vi "oa_TV Time Index Angle (1Chan).vi"(0 "pulse positions":dbl[](array[numeric]), 5 "angle intervals":dbl[](array[numeric]), 7 "revolution":i32, 9 "revolution index":i32, 11 "error in (no error)":errorcluster) -> (4 "pulse positions":dbl[](array[numeric]), 6 "angle":dbl[](array[numeric]), 15 "error out":errorcluster)   [LabVIEW 2017, in "SoundVib_Torsional.lvlib"]
uses:
  <vilib>/addons/Sound and Vibration/Order Analysis/Torsional Vibration/SoundVib_Torsional.lvlib
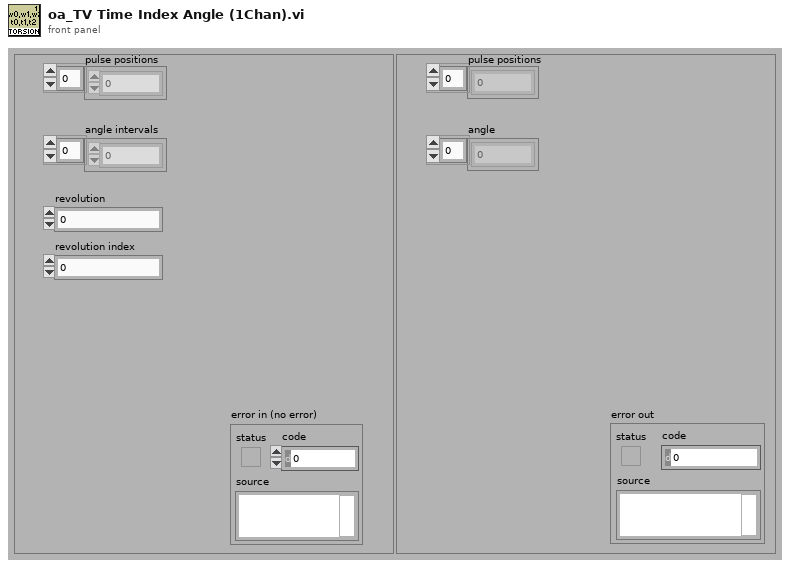
[diagram p1: front panel]
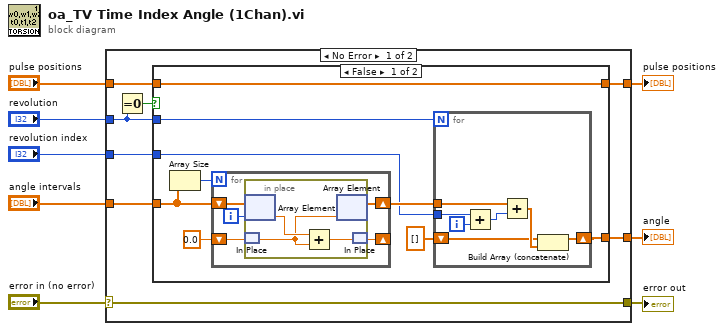
[diagram p0: block diagram]
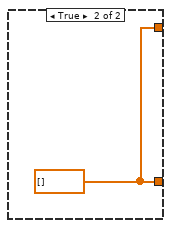
[diagram p2: hidden frame]
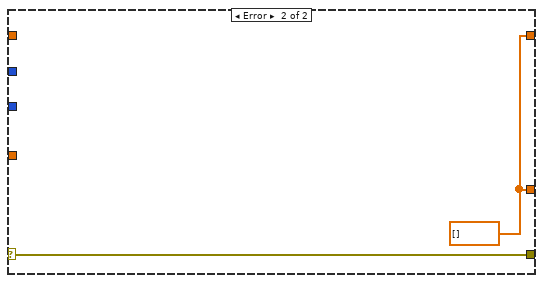
[diagram p3: hidden frame]
diagram:
  n1 = case shown="No Error" "error in (no error)" {
    selector: "error in (no error)" -> [w13 w43]
    tunnel: "angle intervals" -> [w16 _]
    tunnel: "revolution index" -> [w15 _]
    tunnel: [w14 w42] -> w8
    tunnel: [w13 w43] -> w6
    tunnel: "revolution" -> [w10 _]
    tunnel: "pulse positions" -> [w11 _]
    tunnel: [w12 w42] -> w1
    frame No Error {
      n2 = Equal To 0?(x=w10) -> (x = 0?=w9:bool)
      n3 = case shown="False" w9 {
        tunnel: w16 -> [w18 _]
        tunnel: w15 -> [w19 _]
        tunnel: [w23 w41] -> w14
        tunnel: w10 -> [w22 _]
        tunnel: [w21 w41] -> w12
        tunnel: w11 -> [w21 _]
        frame False {
          n4 = Array Size(array=w18) -> (size(s)=w17:i32)
          n5 = for {
            N: w17 -> [_]
            shift-right: [w26] -> _
            shift-left: 0.0 -> [w27]
            shift-right: [w28] -> w20
            shift-left: w18 -> [w30]
            i -> [w29]
            n6 = in-place {
              n7 = in-place-array #1(w30, w29) -> (w33:dbl)
              n8 = in-place-match #2(w27) -> (w31:dbl)
              n9 = Add(x=w33, y=w31) -> (x+y=w32:dbl)
              n10 = in-place-array #1(w31) -> (w28:dbl[])  [unwired: 1 out]
              n11 = in-place-match #2(w32) -> (w26:dbl)
            }
          }
          n12 = for {
            N: w22 -> [_]
            tunnel: w20 -> [w37]
            shift-right: [w39] -> w23
            shift-left: dbl[] [] -> [w38]
            tunnel: w19 -> [w35]
            i -> [w36]
            n13 = Add(x=w35, y=w36) -> (x+y=w34:i32)
            n14 = Add(x=w37, y=w34) -> (x+y=w40:dbl[])
            n15 = Build Array (concatenate)(w38, w40) -> (w39:dbl[])
          }
        }
        frame True {
          w41 = dbl[] [] ("pulse positions")
        }
      }
    }
    frame Error {
      w42 = dbl[] []
    }
  }
  "angle" <- w8
  "error out" <- w6
  "pulse positions" <- w1
